vi "writereport.vi"(10 "Array":T1(array[cluster])) -> ()   [LabVIEW 2012]
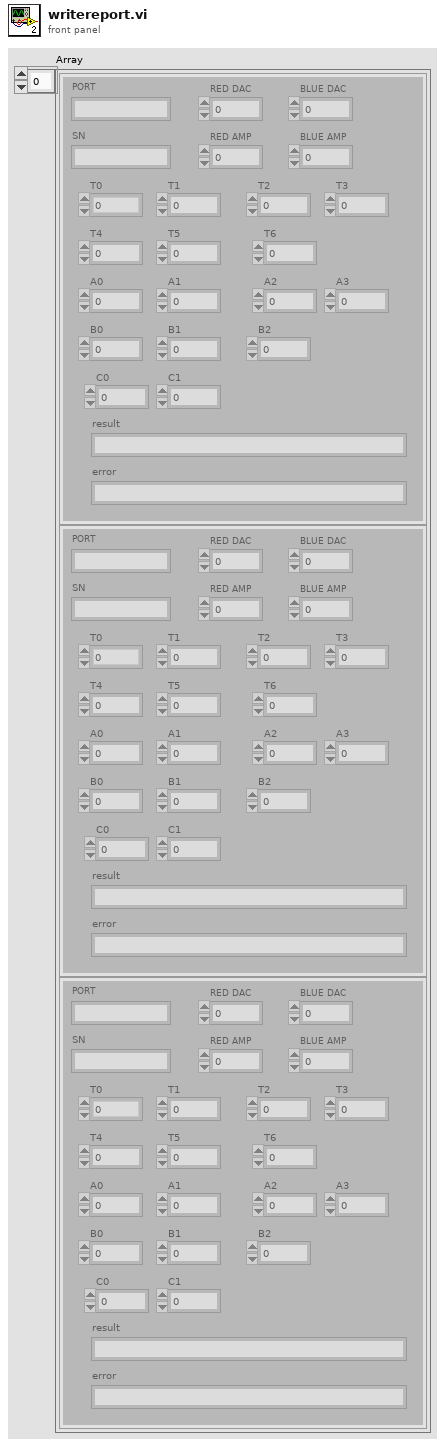
[diagram p1: front panel]
types:
  T1 = cluster{"PORT":string, "SN":string, "RED DAC":dbl, "BLUE DAC":dbl, "RED AMP":dbl, "BLUE AMP":dbl, "T0":dbl, "T1":dbl, "T2":dbl, "T3":dbl, "T4":dbl, "T5":dbl, "T6":dbl, "A0":dbl, "A1":dbl, "A2":dbl, "A3":dbl, "B0":dbl, "B1":dbl, "B2":dbl, "C1":dbl, "C0":dbl, "result":string, "error":string}[]
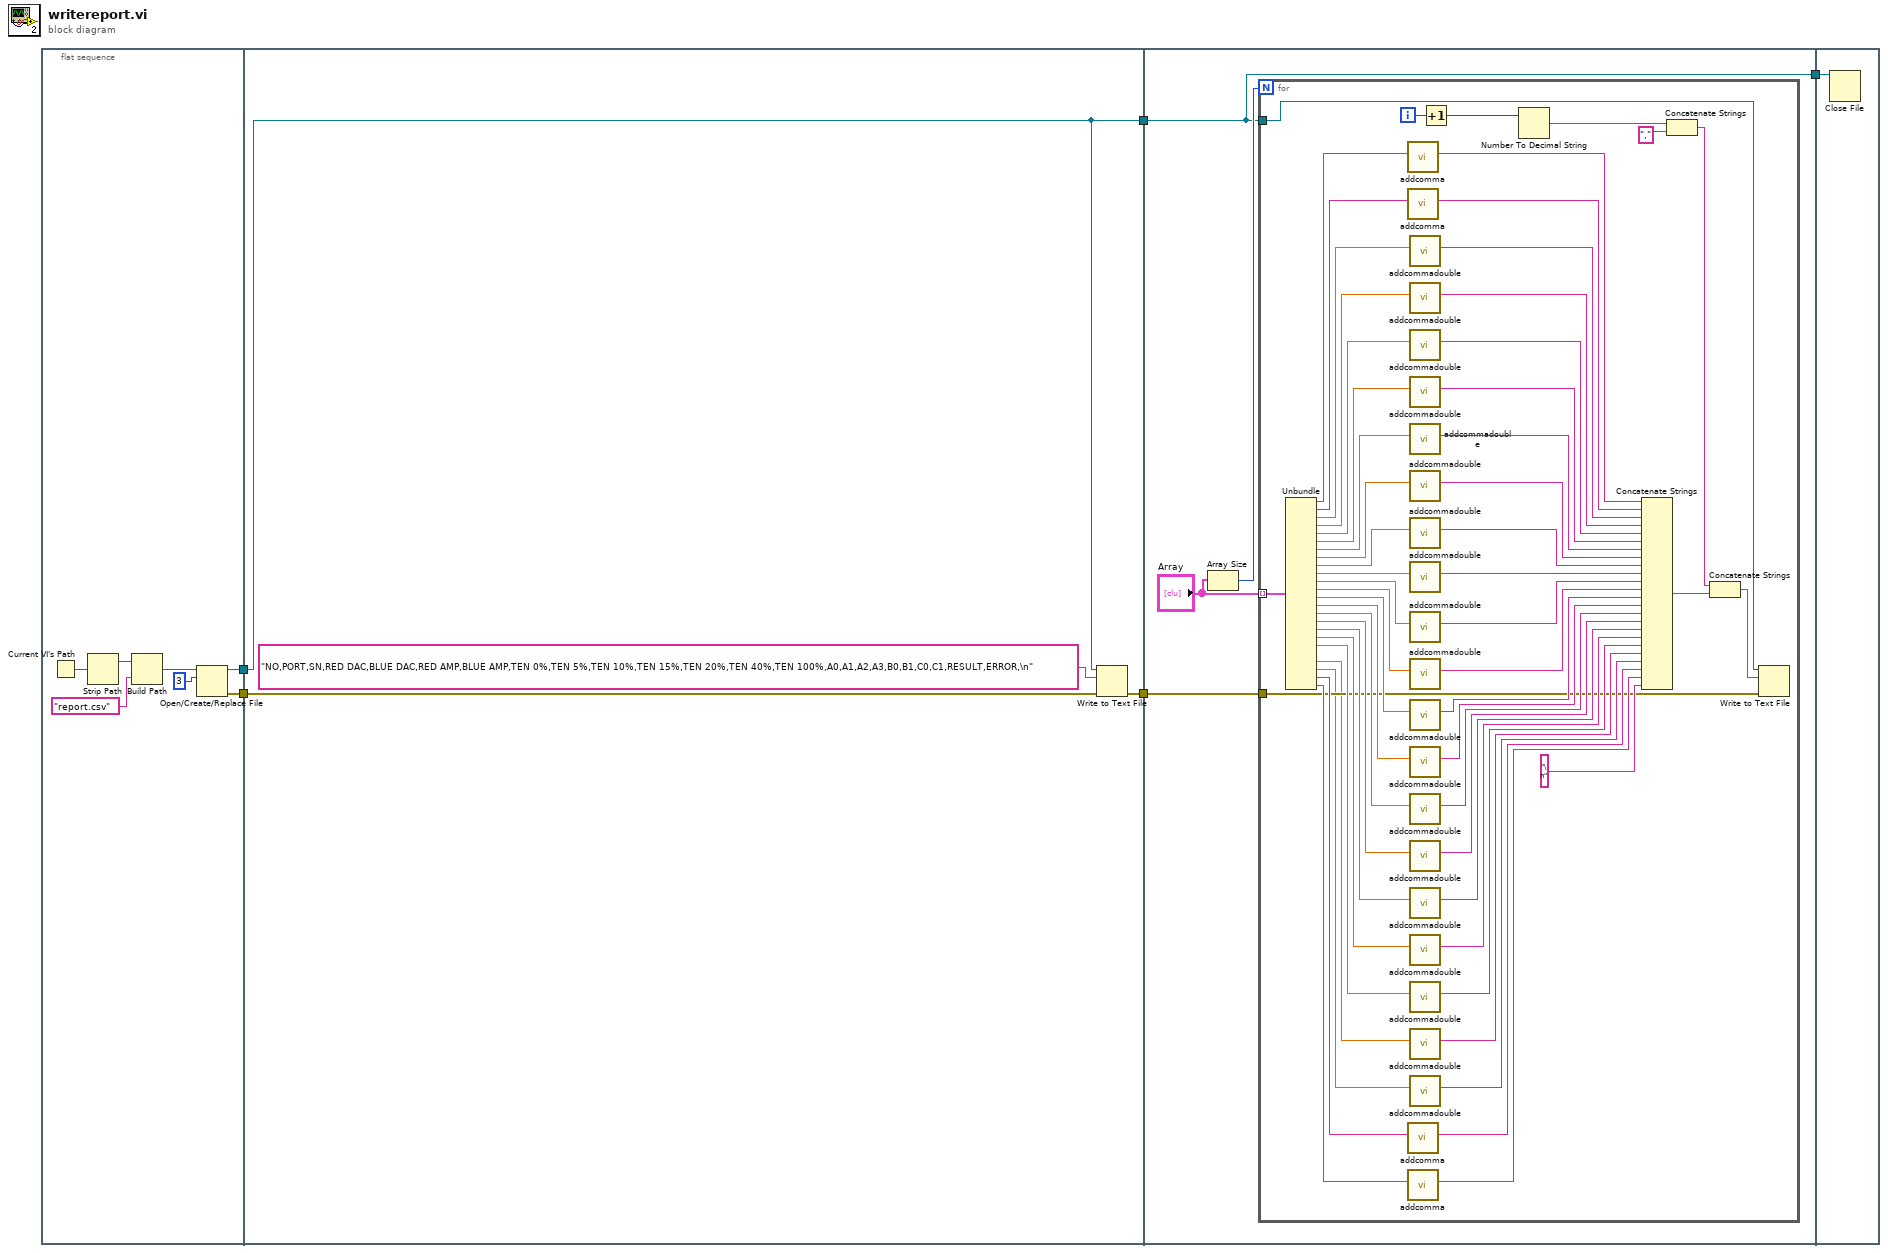
[diagram p0: block diagram]
diagram:
  n1 = flat-sequence {
    tunnel: [w7] -> w5
    tunnel: [w6] -> w4
    tunnel: w5 -> [w14]
    tunnel: w4 -> [w15]
    tunnel: [w14] -> w3
    tunnel: [w13] -> w2
    tunnel: w3 -> [w17]
    tunnel: w2 -> [w18]
    tunnel: [w17] -> w1
    tunnel: w1 -> [w78]
    frame #0 {
      n2 = Current VI's Path() -> (path=w8:path)
      n3 = Strip Path(path=w8) -> (stripped path=w9:path)  [unwired: 1 out]
      n4 = Build Path(base path=w9, name or relative path="report.csv") -> (appended path=w12:path)
      n5 = Open/Create/Replace File(file path (use dialog)=w12, operation (0:open)=3) -> (refnum out=w7:refnum<file>, error out=w6:errorcluster)  [unwired: 4 in, 1 out]
    }
    frame #1 {
      n6 = Write to Text File(file (use dialog)=w14, text="NO,PORT,SN,RED DAC,BLUE DAC,RED AMP,BLUE AMP,TEN 0%,TEN 5%,TEN 10%,TEN 15%,TEN 20%,TEN 40%,TEN 100%,A0,A1,A2,A3,B0,B1,C0,C1,RESULT,ERROR,\n", error in=w15) -> (error out=w13:errorcluster)  [unwired: 1 in, 2 out]
    }
    frame #2 {
      n7 = Array Size(array="Array") -> (size(s)=w20:i32)
      n8 = for {
        N: w20 -> [_]
        tunnel: "Array" -> [w77] mode=indexing
        tunnel: w17 -> [w31]
        tunnel: w18 -> [w30]
        i -> [w24]
        n9 = Unbundle(w77) -> ("PORT"=w73:string, "SN"=w74:string, "RED DAC"=w70:dbl, "BLUE DAC"=w67:dbl, "RED AMP"=w66:dbl, "BLUE AMP"=w64:dbl, "T0"=w62:dbl, "T1"=w60:dbl, "T2"=w58:dbl, "T3"=w55:dbl, "T4"=w54:dbl, "T5"=w51:dbl, "T6"=w50:dbl, "A0"=w47:dbl, "A1"=w46:dbl, "A2"=w43:dbl, "A3"=w42:dbl, "B0"=w40:dbl, "B1"=w38:dbl, "C1"=w22:dbl, "C0"=w21:dbl, "result"=w76:string, "error"=w75:string)  [unwired: 1 out]
        n10 = call "addcomma.vi"("INPUT"=w73) -> ("OUTPUT"=w72:string)  [unwired: 10 in]
        n11 = call "addcomma.vi"("INPUT"=w74) -> ("OUTPUT"=w71:string)  [unwired: 10 in]
        n12 = call "addcomma.vi"("INPUT"=w76) -> ("OUTPUT"=w34:string)  [unwired: 10 in]
        n13 = call "addcomma.vi"("INPUT"=w75) -> ("OUTPUT"=w33:string)  [unwired: 10 in]
        n14 = call "addcommadouble.vi"("input"=w70) -> ("output"=w69:string)  [unwired: 10 in]
        n15 = call "addcommadouble.vi"("input"=w67) -> ("output"=w68:string)  [unwired: 10 in]
        n16 = call "addcommadouble.vi"("input"=w66) -> ("output"=w65:string)  [unwired: 10 in]
        n17 = call "addcommadouble.vi"("input"=w64) -> ("output"=w63:string)  [unwired: 10 in]
        n18 = call "addcommadouble.vi"("input"=w62) -> ("output"=w61:string)  [unwired: 10 in]
        n19 = call "addcommadouble.vi"("input"=w60) -> ("output"=w59:string)  [unwired: 10 in]
        n20 = call "addcommadouble.vi"("input"=w58) -> ("output"=w57:string)  [unwired: 10 in]
        n21 = call "addcommadouble.vi"("input"=w55) -> ("output"=w56:string)  [unwired: 10 in]
        n22 = call "addcommadouble.vi"("input"=w54) -> ("output"=w53:string)  [unwired: 10 in]
        n23 = call "addcommadouble.vi"("input"=w51) -> ("output"=w52:string)  [unwired: 10 in]
        n24 = call "addcommadouble.vi"("input"=w50) -> ("output"=w49:string)  [unwired: 10 in]
        n25 = call "addcommadouble.vi"("input"=w47) -> ("output"=w48:string)  [unwired: 10 in]
        n26 = call "addcommadouble.vi"("input"=w46) -> ("output"=w45:string)  [unwired: 10 in]
        n27 = call "addcommadouble.vi"("input"=w43) -> ("output"=w44:string)  [unwired: 10 in]
        n28 = call "addcommadouble.vi"("input"=w42) -> ("output"=w41:string)  [unwired: 10 in]
        n29 = call "addcommadouble.vi"("input"=w40) -> ("output"=w39:string)  [unwired: 10 in]
        n30 = call "addcommadouble.vi"("input"=w38) -> ("output"=w37:string)  [unwired: 10 in]
        n31 = call "addcommadouble.vi"("input"=w22) -> ("output"=w35:string)  [unwired: 10 in]
        n32 = call "addcommadouble.vi"("input"=w21) -> ("output"=w36:string)  [unwired: 10 in]
        n33 = Increment(x=w24) -> (x+1=w23:i32)
        n34 = Number To Decimal String(number=w23) -> (decimal integer string=w27:string)  [unwired: 1 in]
        n35 = Concatenate Strings(w72, w71, w69, w68, w65, w63, w61, w59, w57, w56, w53, w52, w49, w48, w45, w44, w41, w39, w37, w35, w36, w34, w33, "\n") -> (w29:string)
        n36 = Concatenate Strings(w27, ",") -> (w25:string)
        n37 = Concatenate Strings(w25, w29) -> (w28:string)
        n38 = Write to Text File(file (use dialog)=w31, text=w28, error in=w30) -> ()  [unwired: 1 in, 3 out]
      }
    }
    frame #3 {
      n39 = Close File(refnum=w78) -> ()  [unwired: 1 in, 2 out]
    }
  }
